vi "20TVTI-Set-NV-Manual.vi"(8 "error in (no error)":errorcluster, 10 "VTI Control":T1, 11 "Mercury Reference In":T2) -> (0 "error out":errorcluster)   [LabVIEW 2016]
uses:
  Equipment/Mercury iXX/Public/Controls/Mercury Reference.ctl
  Equipment/Mercury iXX/Public/Controls/Comms Transport Layer.ctl
  Equipment/Mercury iXX/Private/Controls/Query Dynamic Reference.ctl
  S16/VTI-control.ctl
  Equipment/Mercury iXX/Public/Libraries/Temperature/Open/Open Temperature Device.vi
  Global/Global Variables/Data_Display_global.vi
  Equipment/Mercury iXX/Mercury iXX.lvlib
  Equipment/Mercury iXX/Public/Libraries/Temperature.lvlib
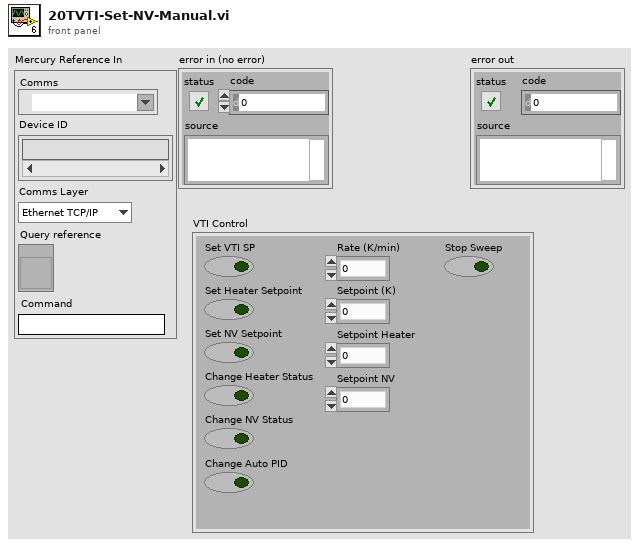
[diagram p1: front panel]
types:
  T1 = typedef "VTI-control.ctl" = cluster{"Set VTI SP":bool, "Change NV Status":bool, "Set NV Setpoint":bool, "Change Heater Status":bool, "Set Heater Setpoint":bool, "Setpoint (K)":dbl, "Rate (K/min)":dbl, "Setpoint Heater":dbl, "Setpoint NV":dbl, "Change Auto PID":bool, "Stop Sweep":bool}
  T2 = typedef "Mercury iXX.lvlib/Mercury Reference.ctl" = cluster{"Comms":refnum<visa-resource-name>, "Device ID":string[], "Comms Layer":T3, "Command":string, "Query reference":T4}
  T3 = typedef "Mercury iXX.lvlib/Comms Transport Layer.ctl" = enum16{"Ethernet TCP/IP", "USB", "ISOBus - RS-232", "GPIB"}
  T4 = typedef "Mercury iXX.lvlib/Query Dynamic Reference.ctl" = refnum<vi>
  T5 = typedef "20TVTI_Cluster.ctl" = cluster{"Temperatur (K)":dbl, "Setpoint (K)":dbl, "Rate (K/min)":dbl, "Heater (%)":dbl, "NV (%)":dbl, "Heater Manual":bool, "NV Manual":bool, "Go to Set":bool, "Pressure":dbl, "Heater SP":dbl, "Valid?":bool, "Set Heater SP":bool, "Set NV SP":bool, "Heater (%) Display":dbl, "NV (%) Display":dbl, "NV Setpoint":dbl, "Change Heater Status":bool, "Change NV Status":bool, "Change Sweep Type":bool}
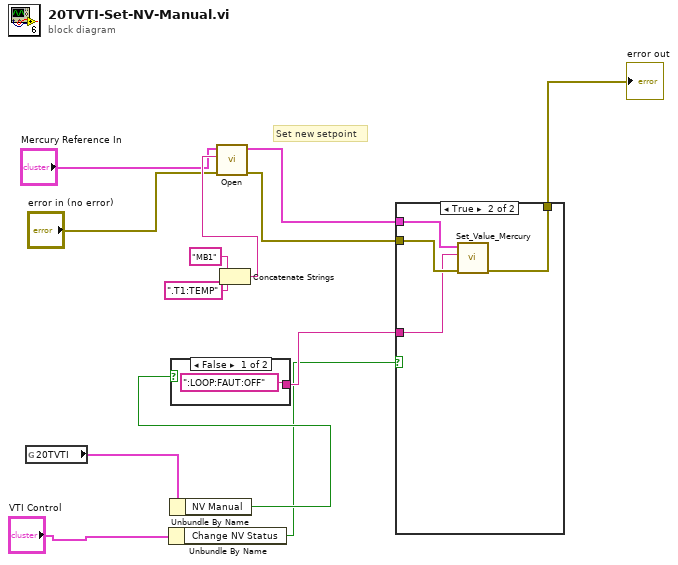
[diagram p0: block diagram]
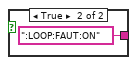
[diagram p2: hidden frame]
diagram:
  # "Set new setpoint"
  n1 = global read "Data_Display_global.vi" "20TVTI"() -> (w11:T5)
  n2 = Unbundle By Name("VTI Control") -> ("Change NV Status"=w2:bool)
  n3 = Unbundle By Name(w11) -> ("NV Manual"=w4:bool)
  n4 = case shown="False" w4 {
    tunnel: [":LOOP:FAUT:OFF" ":LOOP:FAUT:ON"] -> w3
    frame False {
    }
    frame True {
    }
  }
  n5 = Concatenate Strings("MB1", ".T1:TEMP" ("Device Identifier")) -> (w8:string)
  n6 = call-poly "Open.vi"("error in (no error)"="error in (no error)", "Device Identifier"=w8, "Mercury Reference In"="Mercury Reference In") -> ("error out"=w12:errorcluster, "Mercury Reference Out"=w13:T2)  [unwired: 2 in, 5 out]
  n7 = case shown="True" w2 {
    tunnel: w13 -> [_ w20]
    tunnel: w12 -> [w16 w19]
    tunnel: [w16 w18] -> w5
    tunnel: w3 -> [_ w17]
    frame False {
    }
    frame True {
      n8 = call "Set_Value_Mercury.vi"("error in"=w19, "Noun(s)"=w17, "Mercury Reference In"=w20) -> ("error out"=w18:errorcluster)  [unwired: 7 in, 1 out]
    }
  }
  "error out" <- w5
